vi "Invoke BuildTarget.vi"(7 "vi reference":refnum<vi>, 8 "error in (no error)":errorcluster, 11 "BuildItem ref":refnum<vi>) -> (0 "error out":errorcluster, 3 "Generated files":path[](array[path]))   [LabVIEW 2020]
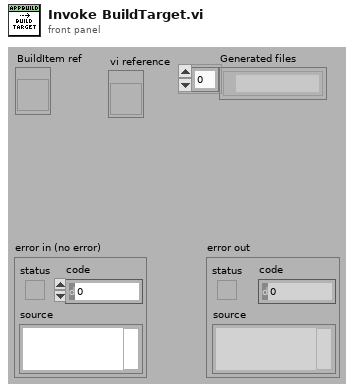
[diagram p1: front panel]
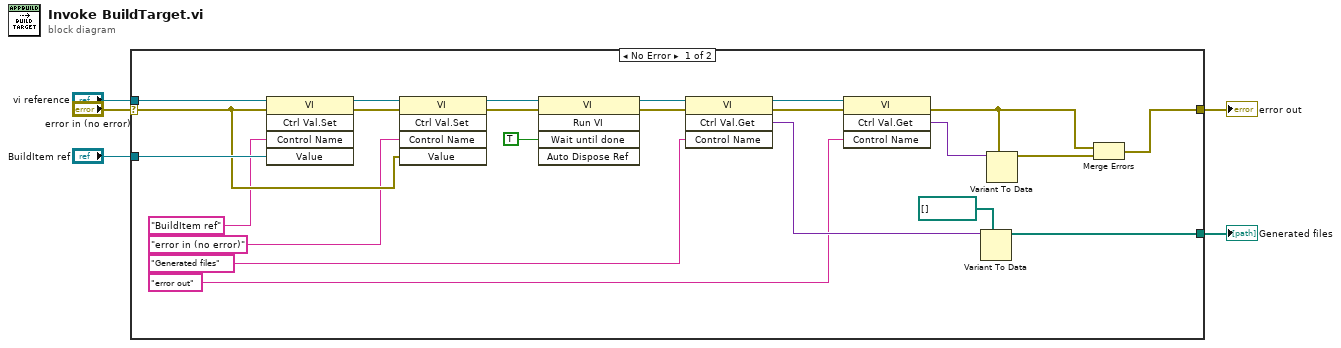
[diagram p0: block diagram]
diagram:
  n1 = case shown="No Error" "error in (no error)" {
    selector: "error in (no error)" -> [w17 w29]
    tunnel: [w6 w29] -> w4
    tunnel: [w12 _] -> w3
    tunnel: "BuildItem ref" -> [w18 _]
    tunnel: "vi reference" -> [w23 _]
    frame No Error {
      n2 = invoke class="VI" method="Ctrl Val.Set"(reference=w23, error in=w17, "Control Name"="BuildItem ref", "Value"=w18) -> (reference out=w22:refnum<vi>, error out=w27:errorcluster)  [unwired: 1 in, 3 out]
      n3 = invoke class="VI" method="Ctrl Val.Set"(reference=w22, error in=w27, "Control Name"="error in (no error)", "Value"=w17) -> (reference out=w21:refnum<vi>, error out=w26:errorcluster)  [unwired: 1 in, 3 out]
      n4 = invoke class="VI" method="Run VI"(reference=w21, error in=w26, "Wait until done"=TRUE ("Wait Until Done")) -> (reference out=w20:refnum<vi>, error out=w25:errorcluster)  [unwired: 2 in, 3 out]
      n5 = invoke class="VI" method="Ctrl Val.Get"(reference=w20, error in=w25, "Control Name"="Generated files") -> (reference out=w19:refnum<vi>, error out=w24:errorcluster, "Get Control Value Variant"=w14:variant)  [unwired: 1 in, 1 out]
      n6 = invoke class="VI" method="Ctrl Val.Get"(reference=w19, error in=w24, "Control Name"="error out") -> (error out=w7:errorcluster, "Get Control Value Variant"=w9:variant)  [unwired: 1 in, 2 out]
      n7 = Variant To Data(type=path[] [] ("Generated Files"), Variant=w14) -> (data=w12:path[])  [unwired: 1 in, 1 out]
      n8 = Variant To Data(type=w7, Variant=w9) -> (data=w8:errorcluster)  [unwired: 1 in, 1 out]
      n9 = Merge Errors(w7, w8) -> (w6:errorcluster)
    }
    frame Error {
    }
  }
  "error out" <- w4
  "Generated files" <- w3
